vi "Data-AnalyzeBooleanData.vi"(8 "error in (no error)":errorcluster, 11 "Meter-Test in":refnum<class "Meter-Test.lvclass">) -> (0 "error out":errorcluster, 2 "Meters That Failed":string, 3 "Meter-Test out":refnum<class "Meter-Test.lvclass">, 5 "Meter Test Passed or Failed":bool)   [LabVIEW 2013, in "Meter-Test.lvclass"]
uses:
  Meter-Test.lvclass
  Meter-Test.lvclass/Meter-Test.ctl
  <userlib>/_OpenG.lib/array/array.llb/Search 1D Array (Boolean)__ogtk.vi
  <userlib>/_OpenG.lib/array/array.llb/Remove Duplicates from 1D Array (I32)__ogtk.vi
  <userlib>/_OpenG.lib/array/array.llb/Empty 1D Array (I32)__ogtk.vi
  <userlib>/_OpenG.lib/array/array.llb/Index 1D Array Elements (Boolean)__ogtk.vi
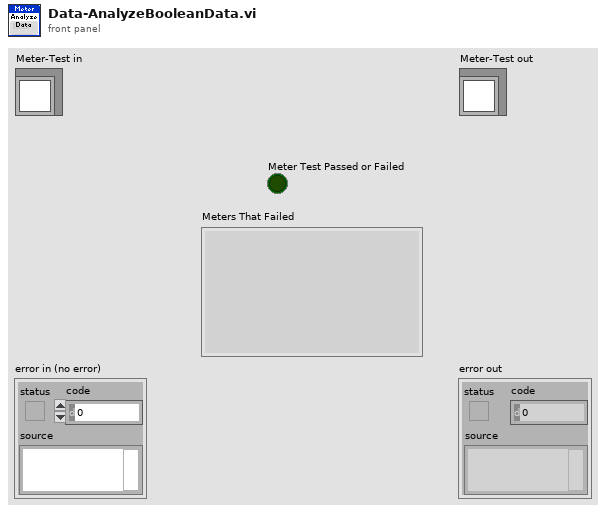
[diagram p1: front panel]
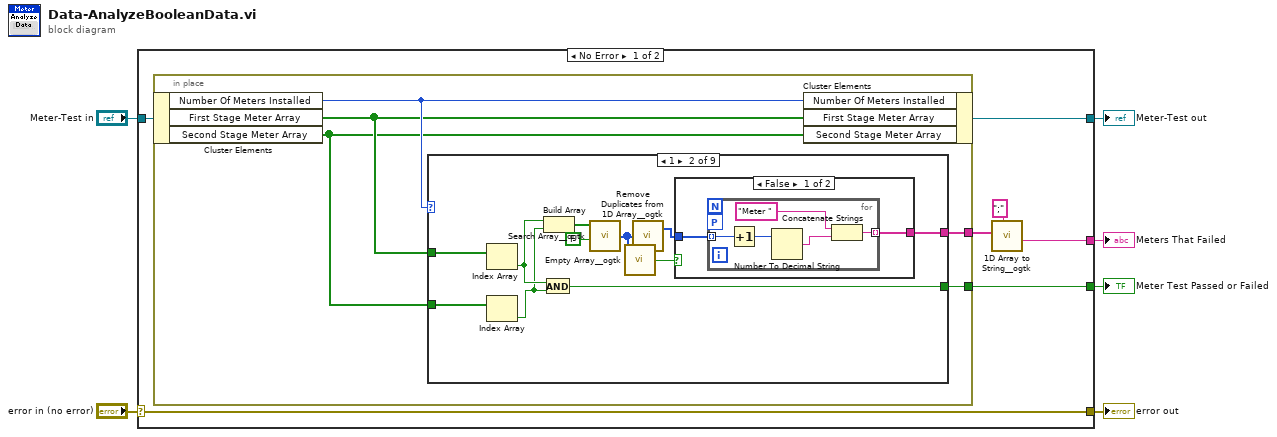
[diagram p0: block diagram]
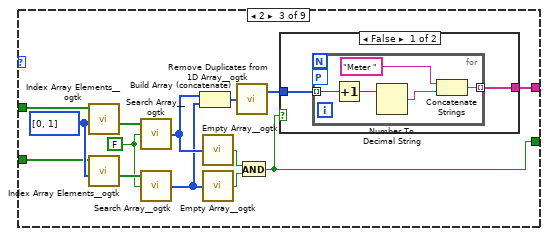
[diagram p4: hidden frame]
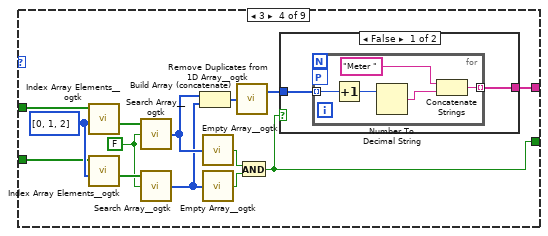
[diagram p6: hidden frame]
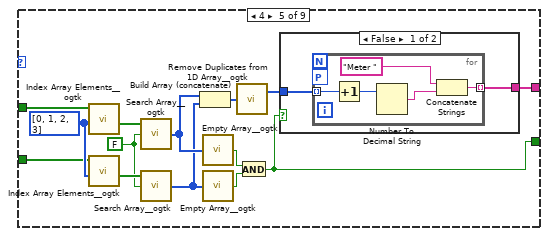
[diagram p8: hidden frame]
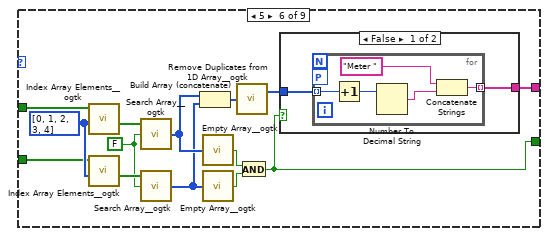
[diagram p10: hidden frame]
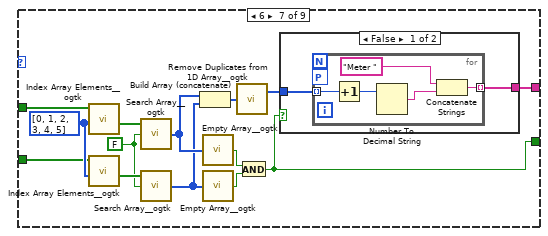
[diagram p12: hidden frame]
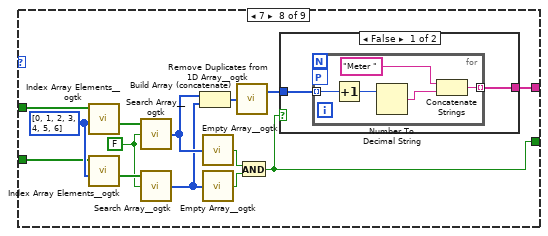
[diagram p14: hidden frame]
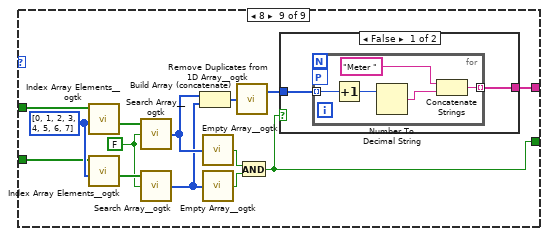
[diagram p16: hidden frame]
diagram:
  n1 = case shown="No Error" "error in (no error)" {
    selector: "error in (no error)" -> [w13 w185]
    tunnel: [w13 w185] -> w5
    tunnel: [w7 w184] -> w3
    tunnel: "Meter-Test in" -> [w8 w184]
    tunnel: [w12 _] -> w2
    tunnel: [w9 _] -> w1
    frame No Error {
      n2 = in-place {
        in-place-border: [w17] -> w12
        in-place-border: [w16] -> w11
        n3 = in-place-cluster #1(w8) -> ("Number Of Meters Installed"=w18:i32, "First Stage Meter Array"=w15:bool[], "Second Stage Meter Array"=w14:bool[])
        n4 = case shown="1" w18 {
          tunnel: w15 -> [_ w29 w49 w70 w91 w112 w133 w154 w175]
          tunnel: w14 -> [_ w28 w48 w69 w90 w111 w132 w153 w174]
          tunnel: [_ w27 w37 w58 w79 w100 w121 w142 w163] -> w17
          tunnel: [_ w21 w44 w65 w86 w107 w128 w149 w170] -> w16
          frame 0, Default {
          }
          frame 1 {
            n5 = Index Array(array=w29) -> (element=w26:bool)  [unwired: 1 in]
            n6 = Index Array(array=w28) -> (element=w25:bool)  [unwired: 1 in]
            n7 = And(x=w26, y=w25) -> (x .and. y?=w27:bool)
            n8 = Build Array(w26, w25) -> (w24:bool[])
            n9 = call-poly <userlib>:"Search Array__ogtk.vi"("Array"=w24, "Element Data"=FALSE) -> ("Indices of Elements"=w20:i32[])  [unwired: 7 in]
            n10 = call-poly <userlib>:"Empty Array__ogtk.vi"("Array"=w20) -> ("Empty Array?"=w22:bool)  [unwired: 8 in]
            n11 = call-poly <userlib>:"Remove Duplicates from 1D Array__ogtk.vi"("Input Array"=w20) -> ("Output Array"=w19:i32[])  [unwired: 1 out]
            n12 = case shown="False" w22 {
              tunnel: w19 -> [w31 _]
              tunnel: [w30 _] -> w21
              frame False {
                n13 = for {
                  tunnel: w31 -> [w36] mode=indexing
                  tunnel: [w32] -> w30 mode=indexing
                  workers-P: _ -> [_]
                  n14 = Increment(x=w36) -> (x+1=w35:i32)
                  n15 = Number To Decimal String(number=w35) -> (decimal integer string=w34:string)  [unwired: 1 in]
                  n16 = Concatenate Strings("Meter ", w34) -> (w32:string)
                }
              }
              frame True {
              }
            }
          }
          frame 2 {
            w45 = FALSE
            w50 = i32[] [0, 1] ("indices")
            n17 = call-poly <userlib>:"Index Array Elements__ogtk.vi"("indices"=w50, "array"=w49) -> ("elements"=w47:bool[])  [unwired: 9 in]
            n18 = call-poly <userlib>:"Index Array Elements__ogtk.vi"("indices"=w50, "array"=w48) -> ("elements"=w46:bool[])  [unwired: 9 in]
            n19 = call-poly <userlib>:"Search Array__ogtk.vi"("Array"=w47, "Element Data"=w45) -> ("Indices of Elements"=w43:i32[])  [unwired: 7 in]
            n20 = call-poly <userlib>:"Search Array__ogtk.vi"("Array"=w46, "Element Data"=w45) -> ("Indices of Elements"=w42:i32[])  [unwired: 7 in]
            n21 = Build Array (concatenate)(w43, w42) -> (w41:i32[])
            n22 = call-poly <userlib>:"Empty Array__ogtk.vi"("Array"=w43) -> ("Empty Array?"=w39:bool)  [unwired: 8 in]
            n23 = call-poly <userlib>:"Empty Array__ogtk.vi"("Array"=w42) -> ("Empty Array?"=w38:bool)  [unwired: 8 in]
            n24 = call-poly <userlib>:"Remove Duplicates from 1D Array__ogtk.vi"("Input Array"=w41) -> ("Output Array"=w40:i32[])  [unwired: 1 out]
            n25 = And(x=w39, y=w38) -> (x .and. y?=w37:bool)
            n26 = case shown="False" w37 {
              tunnel: [w52 _] -> w44
              tunnel: w40 -> [w51 _]
              frame False {
                n27 = for {
                  tunnel: [w54] -> w52 mode=indexing
                  tunnel: w51 -> [w53] mode=indexing
                  workers-P: _ -> [_]
                  n28 = Increment(x=w53) -> (x+1=w57:i32)
                  n29 = Number To Decimal String(number=w57) -> (decimal integer string=w56:string)  [unwired: 1 in]
                  n30 = Concatenate Strings("Meter ", w56) -> (w54:string)
                }
              }
              frame True {
              }
            }
          }
          frame 3 {
            w66 = FALSE
            w71 = i32[] [0, 1, 2] ("indices")
            n31 = call-poly <userlib>:"Index Array Elements__ogtk.vi"("indices"=w71, "array"=w70) -> ("elements"=w68:bool[])  [unwired: 9 in]
            n32 = call-poly <userlib>:"Index Array Elements__ogtk.vi"("indices"=w71, "array"=w69) -> ("elements"=w67:bool[])  [unwired: 9 in]
            n33 = call-poly <userlib>:"Search Array__ogtk.vi"("Array"=w68, "Element Data"=w66) -> ("Indices of Elements"=w64:i32[])  [unwired: 7 in]
            n34 = call-poly <userlib>:"Search Array__ogtk.vi"("Array"=w67, "Element Data"=w66) -> ("Indices of Elements"=w63:i32[])  [unwired: 7 in]
            n35 = Build Array (concatenate)(w64, w63) -> (w62:i32[])
            n36 = call-poly <userlib>:"Empty Array__ogtk.vi"("Array"=w64) -> ("Empty Array?"=w60:bool)  [unwired: 8 in]
            n37 = call-poly <userlib>:"Empty Array__ogtk.vi"("Array"=w63) -> ("Empty Array?"=w59:bool)  [unwired: 8 in]
            n38 = call-poly <userlib>:"Remove Duplicates from 1D Array__ogtk.vi"("Input Array"=w62) -> ("Output Array"=w61:i32[])  [unwired: 1 out]
            n39 = And(x=w60, y=w59) -> (x .and. y?=w58:bool)
            n40 = case shown="False" w58 {
              tunnel: [w73 _] -> w65
              tunnel: w61 -> [w72 _]
              frame False {
                n41 = for {
                  tunnel: [w75] -> w73 mode=indexing
                  tunnel: w72 -> [w74] mode=indexing
                  workers-P: _ -> [_]
                  n42 = Increment(x=w74) -> (x+1=w78:i32)
                  n43 = Number To Decimal String(number=w78) -> (decimal integer string=w77:string)  [unwired: 1 in]
                  n44 = Concatenate Strings("Meter ", w77) -> (w75:string)
                }
              }
              frame True {
              }
            }
          }
          frame 4 {
            w87 = FALSE
            w92 = i32[] [0, 1, 2, 3] ("indices")
            n45 = call-poly <userlib>:"Index Array Elements__ogtk.vi"("indices"=w92, "array"=w91) -> ("elements"=w89:bool[])  [unwired: 9 in]
            n46 = call-poly <userlib>:"Index Array Elements__ogtk.vi"("indices"=w92, "array"=w90) -> ("elements"=w88:bool[])  [unwired: 9 in]
            n47 = call-poly <userlib>:"Search Array__ogtk.vi"("Array"=w89, "Element Data"=w87) -> ("Indices of Elements"=w85:i32[])  [unwired: 7 in]
            n48 = call-poly <userlib>:"Search Array__ogtk.vi"("Array"=w88, "Element Data"=w87) -> ("Indices of Elements"=w84:i32[])  [unwired: 7 in]
            n49 = Build Array (concatenate)(w85, w84) -> (w83:i32[])
            n50 = call-poly <userlib>:"Empty Array__ogtk.vi"("Array"=w85) -> ("Empty Array?"=w81:bool)  [unwired: 8 in]
            n51 = call-poly <userlib>:"Empty Array__ogtk.vi"("Array"=w84) -> ("Empty Array?"=w80:bool)  [unwired: 8 in]
            n52 = call-poly <userlib>:"Remove Duplicates from 1D Array__ogtk.vi"("Input Array"=w83) -> ("Output Array"=w82:i32[])  [unwired: 1 out]
            n53 = And(x=w81, y=w80) -> (x .and. y?=w79:bool)
            n54 = case shown="False" w79 {
              tunnel: [w94 _] -> w86
              tunnel: w82 -> [w93 _]
              frame False {
                n55 = for {
                  tunnel: [w96] -> w94 mode=indexing
                  tunnel: w93 -> [w95] mode=indexing
                  workers-P: _ -> [_]
                  n56 = Increment(x=w95) -> (x+1=w99:i32)
                  n57 = Number To Decimal String(number=w99) -> (decimal integer string=w98:string)  [unwired: 1 in]
                  n58 = Concatenate Strings("Meter ", w98) -> (w96:string)
                }
              }
              frame True {
              }
            }
          }
          frame 5 {
            w108 = FALSE
            w113 = i32[] [0, 1, 2, 3, 4] ("indices")
            n59 = call-poly <userlib>:"Index Array Elements__ogtk.vi"("indices"=w113, "array"=w112) -> ("elements"=w110:bool[])  [unwired: 9 in]
            n60 = call-poly <userlib>:"Index Array Elements__ogtk.vi"("indices"=w113, "array"=w111) -> ("elements"=w109:bool[])  [unwired: 9 in]
            n61 = call-poly <userlib>:"Search Array__ogtk.vi"("Array"=w110, "Element Data"=w108) -> ("Indices of Elements"=w106:i32[])  [unwired: 7 in]
            n62 = call-poly <userlib>:"Search Array__ogtk.vi"("Array"=w109, "Element Data"=w108) -> ("Indices of Elements"=w105:i32[])  [unwired: 7 in]
            n63 = Build Array (concatenate)(w106, w105) -> (w104:i32[])
            n64 = call-poly <userlib>:"Empty Array__ogtk.vi"("Array"=w106) -> ("Empty Array?"=w102:bool)  [unwired: 8 in]
            n65 = call-poly <userlib>:"Empty Array__ogtk.vi"("Array"=w105) -> ("Empty Array?"=w101:bool)  [unwired: 8 in]
            n66 = call-poly <userlib>:"Remove Duplicates from 1D Array__ogtk.vi"("Input Array"=w104) -> ("Output Array"=w103:i32[])  [unwired: 1 out]
            n67 = And(x=w102, y=w101) -> (x .and. y?=w100:bool)
            n68 = case shown="False" w100 {
              tunnel: [w115 _] -> w107
              tunnel: w103 -> [w114 _]
              frame False {
                n69 = for {
                  tunnel: [w117] -> w115 mode=indexing
                  tunnel: w114 -> [w116] mode=indexing
                  workers-P: _ -> [_]
                  n70 = Increment(x=w116) -> (x+1=w120:i32)
                  n71 = Number To Decimal String(number=w120) -> (decimal integer string=w119:string)  [unwired: 1 in]
                  n72 = Concatenate Strings("Meter ", w119) -> (w117:string)
                }
              }
              frame True {
              }
            }
          }
          frame 6 {
            w129 = FALSE
            w134 = i32[] [0, 1, 2, 3, 4, 5] ("indices")
            n73 = call-poly <userlib>:"Index Array Elements__ogtk.vi"("indices"=w134, "array"=w133) -> ("elements"=w131:bool[])  [unwired: 9 in]
            n74 = call-poly <userlib>:"Index Array Elements__ogtk.vi"("indices"=w134, "array"=w132) -> ("elements"=w130:bool[])  [unwired: 9 in]
            n75 = call-poly <userlib>:"Search Array__ogtk.vi"("Array"=w131, "Element Data"=w129) -> ("Indices of Elements"=w127:i32[])  [unwired: 7 in]
            n76 = call-poly <userlib>:"Search Array__ogtk.vi"("Array"=w130, "Element Data"=w129) -> ("Indices of Elements"=w126:i32[])  [unwired: 7 in]
            n77 = Build Array (concatenate)(w127, w126) -> (w125:i32[])
            n78 = call-poly <userlib>:"Empty Array__ogtk.vi"("Array"=w127) -> ("Empty Array?"=w123:bool)  [unwired: 8 in]
            n79 = call-poly <userlib>:"Empty Array__ogtk.vi"("Array"=w126) -> ("Empty Array?"=w122:bool)  [unwired: 8 in]
            n80 = call-poly <userlib>:"Remove Duplicates from 1D Array__ogtk.vi"("Input Array"=w125) -> ("Output Array"=w124:i32[])  [unwired: 1 out]
            n81 = And(x=w123, y=w122) -> (x .and. y?=w121:bool)
            n82 = case shown="False" w121 {
              tunnel: [w136 _] -> w128
              tunnel: w124 -> [w135 _]
              frame False {
                n83 = for {
                  tunnel: [w138] -> w136 mode=indexing
                  tunnel: w135 -> [w137] mode=indexing
                  workers-P: _ -> [_]
                  n84 = Increment(x=w137) -> (x+1=w141:i32)
                  n85 = Number To Decimal String(number=w141) -> (decimal integer string=w140:string)  [unwired: 1 in]
                  n86 = Concatenate Strings("Meter ", w140) -> (w138:string)
                }
              }
              frame True {
              }
            }
          }
          frame 7 {
            w150 = FALSE
            w155 = i32[] [0, 1, 2, 3, 4, 5, 6] ("indices")
            n87 = call-poly <userlib>:"Index Array Elements__ogtk.vi"("indices"=w155, "array"=w154) -> ("elements"=w152:bool[])  [unwired: 9 in]
            n88 = call-poly <userlib>:"Index Array Elements__ogtk.vi"("indices"=w155, "array"=w153) -> ("elements"=w151:bool[])  [unwired: 9 in]
            n89 = call-poly <userlib>:"Search Array__ogtk.vi"("Array"=w152, "Element Data"=w150) -> ("Indices of Elements"=w148:i32[])  [unwired: 7 in]
            n90 = call-poly <userlib>:"Search Array__ogtk.vi"("Array"=w151, "Element Data"=w150) -> ("Indices of Elements"=w147:i32[])  [unwired: 7 in]
            n91 = Build Array (concatenate)(w148, w147) -> (w146:i32[])
            n92 = call-poly <userlib>:"Empty Array__ogtk.vi"("Array"=w148) -> ("Empty Array?"=w144:bool)  [unwired: 8 in]
            n93 = call-poly <userlib>:"Empty Array__ogtk.vi"("Array"=w147) -> ("Empty Array?"=w143:bool)  [unwired: 8 in]
            n94 = call-poly <userlib>:"Remove Duplicates from 1D Array__ogtk.vi"("Input Array"=w146) -> ("Output Array"=w145:i32[])  [unwired: 1 out]
            n95 = And(x=w144, y=w143) -> (x .and. y?=w142:bool)
            n96 = case shown="False" w142 {
              tunnel: [w157 _] -> w149
              tunnel: w145 -> [w156 _]
              frame False {
                n97 = for {
                  tunnel: [w159] -> w157 mode=indexing
                  tunnel: w156 -> [w158] mode=indexing
                  workers-P: _ -> [_]
                  n98 = Increment(x=w158) -> (x+1=w162:i32)
                  n99 = Number To Decimal String(number=w162) -> (decimal integer string=w161:string)  [unwired: 1 in]
                  n100 = Concatenate Strings("Meter ", w161) -> (w159:string)
                }
              }
              frame True {
              }
            }
          }
          frame 8 {
            w171 = FALSE
            w176 = i32[] [0, 1, 2, 3, 4, 5, 6, 7] ("indices")
            n101 = call-poly <userlib>:"Index Array Elements__ogtk.vi"("indices"=w176, "array"=w175) -> ("elements"=w173:bool[])  [unwired: 9 in]
            n102 = call-poly <userlib>:"Index Array Elements__ogtk.vi"("indices"=w176, "array"=w174) -> ("elements"=w172:bool[])  [unwired: 9 in]
            n103 = call-poly <userlib>:"Search Array__ogtk.vi"("Array"=w173, "Element Data"=w171) -> ("Indices of Elements"=w169:i32[])  [unwired: 7 in]
            n104 = call-poly <userlib>:"Search Array__ogtk.vi"("Array"=w172, "Element Data"=w171) -> ("Indices of Elements"=w168:i32[])  [unwired: 7 in]
            n105 = Build Array (concatenate)(w169, w168) -> (w167:i32[])
            n106 = call-poly <userlib>:"Empty Array__ogtk.vi"("Array"=w169) -> ("Empty Array?"=w165:bool)  [unwired: 8 in]
            n107 = call-poly <userlib>:"Empty Array__ogtk.vi"("Array"=w168) -> ("Empty Array?"=w164:bool)  [unwired: 8 in]
            n108 = call-poly <userlib>:"Remove Duplicates from 1D Array__ogtk.vi"("Input Array"=w167) -> ("Output Array"=w166:i32[])  [unwired: 1 out]
            n109 = And(x=w165, y=w164) -> (x .and. y?=w163:bool)
            n110 = case shown="False" w163 {
              tunnel: [w178 _] -> w170
              tunnel: w166 -> [w177 _]
              frame False {
                n111 = for {
                  tunnel: [w180] -> w178 mode=indexing
                  tunnel: w177 -> [w179] mode=indexing
                  workers-P: _ -> [_]
                  n112 = Increment(x=w179) -> (x+1=w183:i32)
                  n113 = Number To Decimal String(number=w183) -> (decimal integer string=w182:string)  [unwired: 1 in]
                  n114 = Concatenate Strings("Meter ", w182) -> (w180:string)
                }
              }
              frame True {
              }
            }
          }
        }
        n115 = in-place-cluster #1("Number Of Meters Installed"=w18, "First Stage Meter Array"=w15, "Second Stage Meter Array"=w14) -> (w7:refnum<class "Meter-Test.lvclass">)
      }
      n116 = call <userlib>:"1D Array to String__ogtk.vi"("delimiter (Tab)"=";", "Array of Strings"=w11) -> ("delimited string"=w9:string)  [unwired: 9 in]
    }
    frame Error {
    }
  }
  "error out" <- w5
  "Meter-Test out" <- w3
  "Meter Test Passed or Failed" <- w2
  "Meters That Failed" <- w1
